vi "aptControl.vi"() -> (0 "Moving":bool, 3 "Current Position":sgl)   [LabVIEW 2010]
uses:
  <vilib>/DAQmx/write.llb/DAQmx Write (Digital 1D Bool 1Chan 1Samp).vi
  <vilib>/DAQmx/read.llb/DAQmx Read (Analog Wfm 1Chan NSamp).vi
  <vilib>/DAQmx/write.llb/DAQmx Write (Analog Wfm 1Chan NSamp).vi
  <vilib>/daqmx/miscellaneous.llb/DAQmx Fill In Error Info.vi
  <vilib>/Utility/file.llb/Write To Spreadsheet File (DBL).vi
  <vilib>/Utility/file.llb/Read From Spreadsheet File (DBL).vi
  <vilib>/gmath/NI_Gmath.lvlib
  <vilib>/Analysis/NI_AALBase.lvlib
panel:
  out "Scaner":string
  in  "Tab Control":enum32{"Control", "Curve", "Calibrate"}(tab)
  out "Es. Power (mW)":dbl format="%#.0f"
  in  "Possition (0:360)":dbl format="%#.2f"
  in  "Up":bool
  in  "Down":bool
  in  "Mirror\nOverride":bool
  in  "Galvo":bool=TRUE caption="AOD"
  in  "Lens":u16(ring)=10 items=["10X"=10, "20X"=20, "25X"=25, "16X"=16, "60X"=60]
  out "Out of range":bool
  in  "Home":bool
  in  "stop":bool
  out "Calibration Used":string
  out "Curve":cluster{"all rows":dbl[], "all rows":dbl[]}(graph)
  out "Curve 2":cluster{i32[], i32[]}(graph)
  in  "Start Calibration":bool
  in  "WaveLengths":dbl[](array[numeric])=[800.0, 890.0]
  out "Finished":bool
  in  "quit":bool
  out "Remaining min":dbl format="%#.2f"
  out "Acquiring":bool
  out "Waiting":bool
  out "Moving 2":bool
  in  "Repetitions":dbl=1.0
  in  "Step Size":dbl=4.0
  out "Current mW":dbl format="%#.0f"
  out "Old possition":sgl
  in  "MG17Motor 2":refnum<k7>(container)
  out "MinPos":sgl
  out "MaxPos":sgl
  in  "Target Position":dbl
  in  "MG17Motor":refnum<k7>(container)
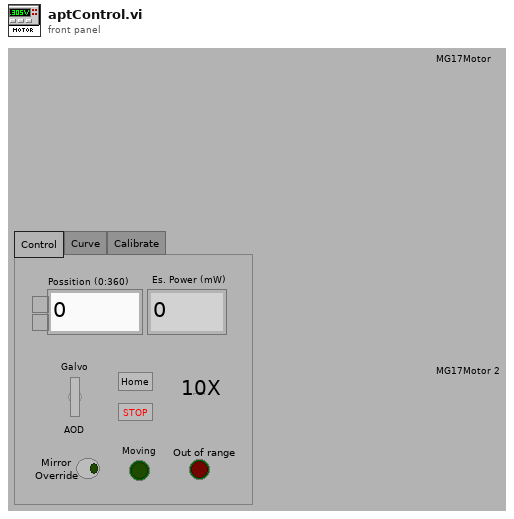
[diagram p1: front panel]
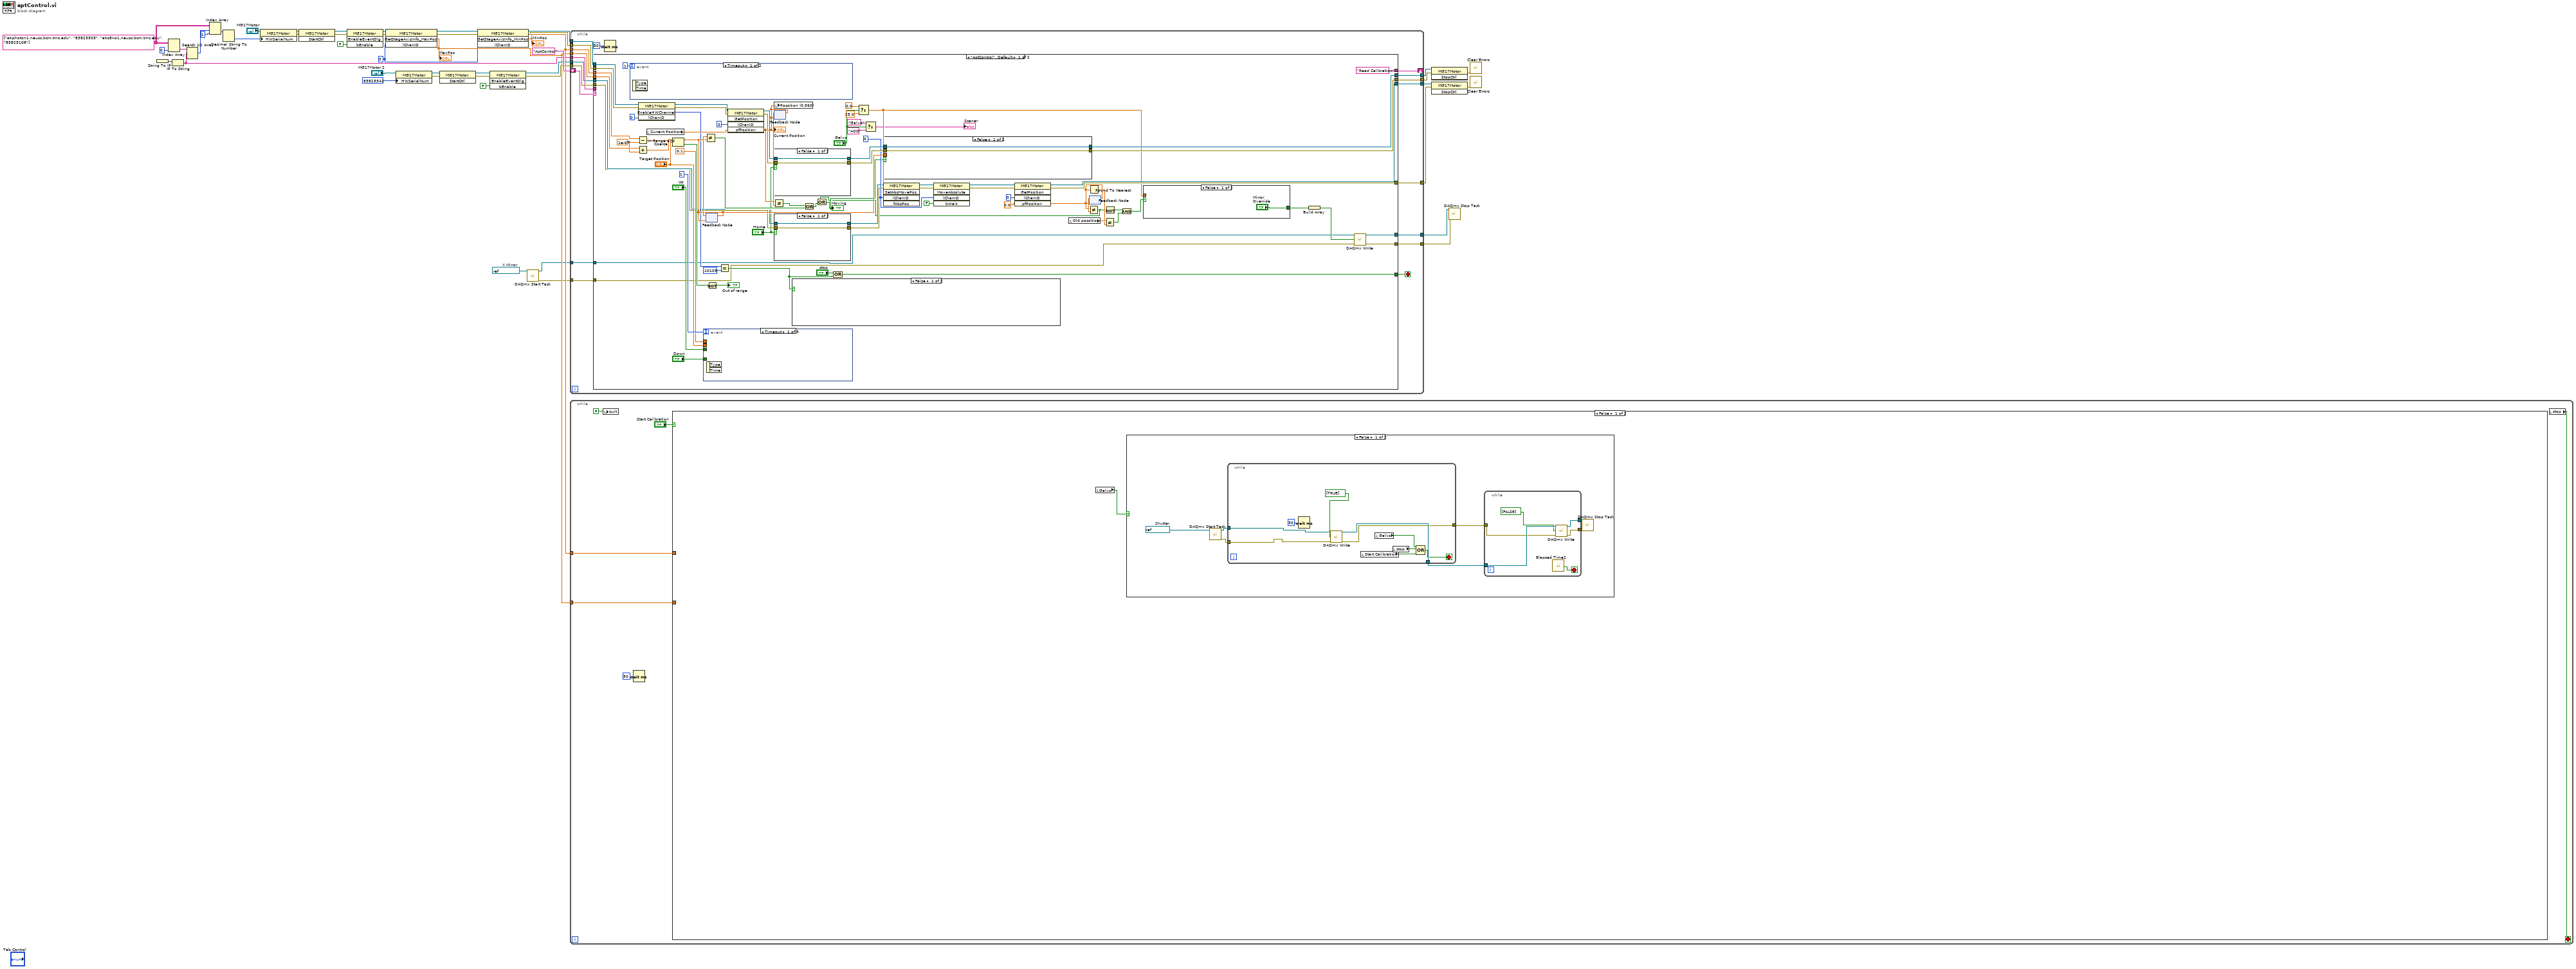
[diagram p0: block diagram]
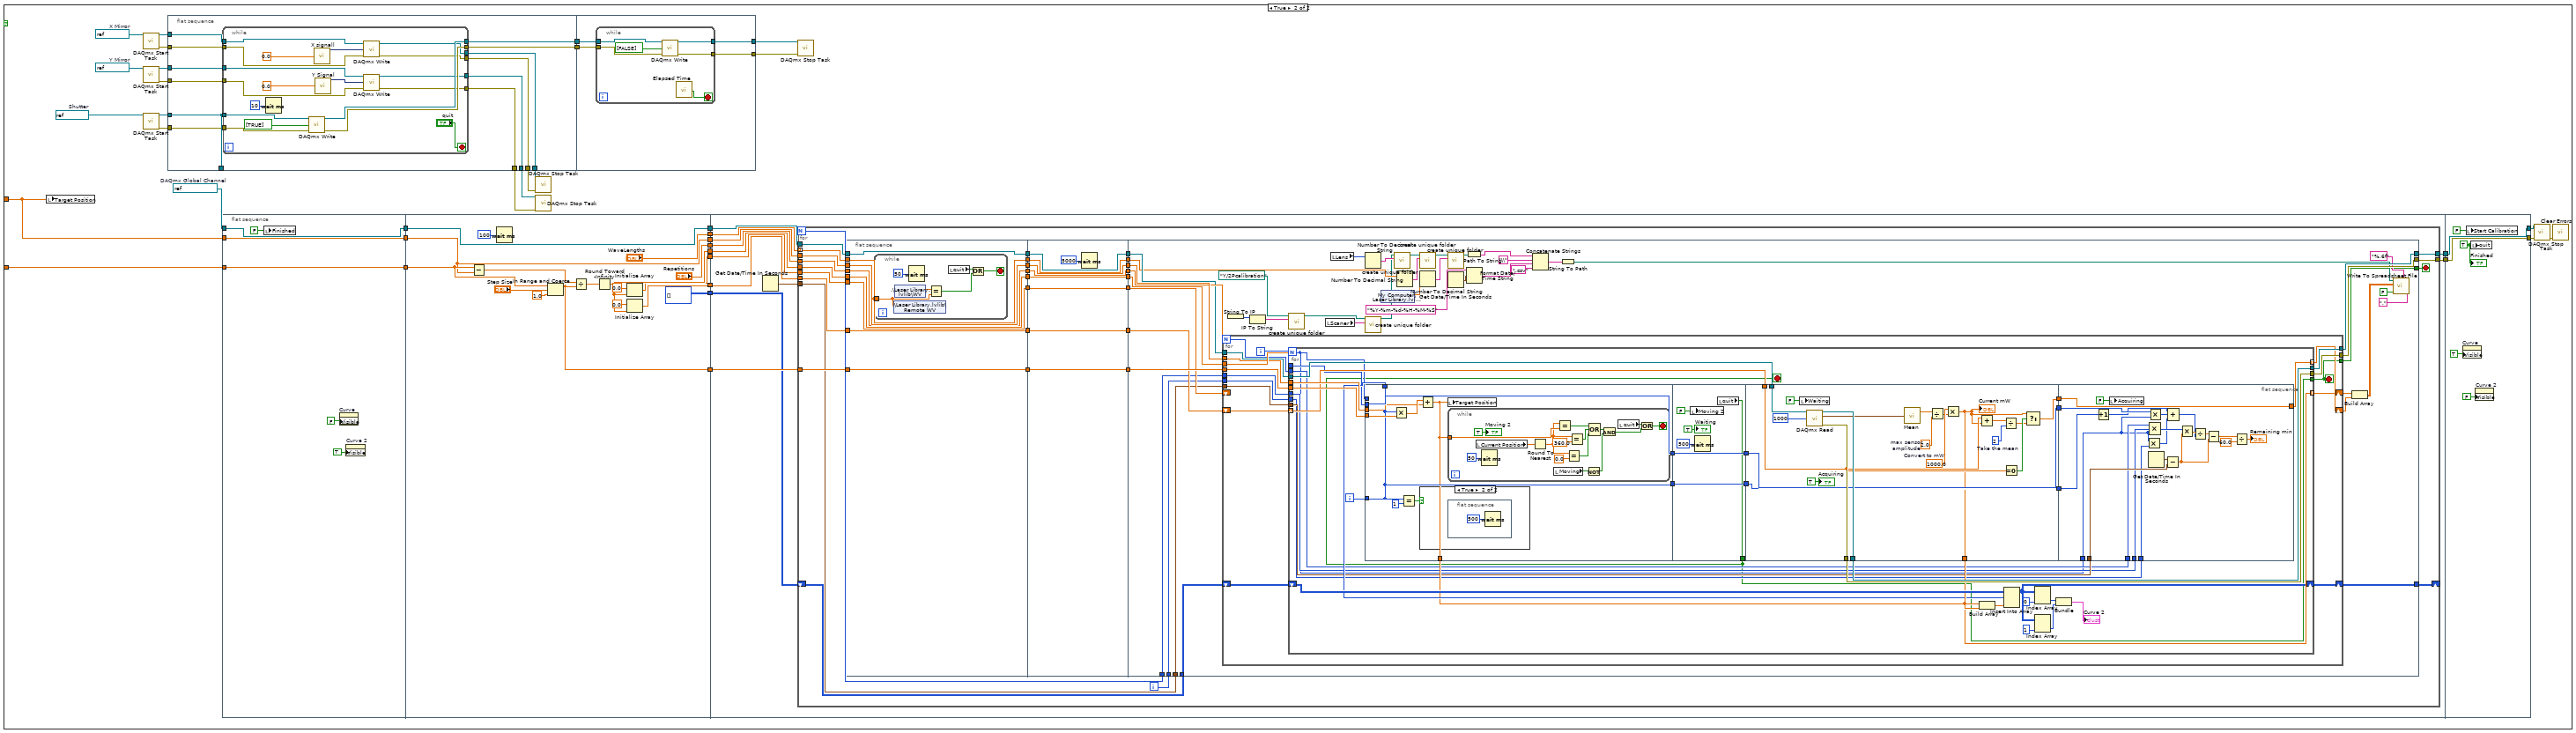
[diagram p3: hidden frame]
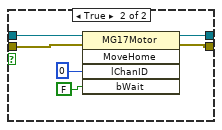
[diagram p5: hidden frame]
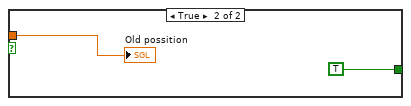
[diagram p6: hidden frame]
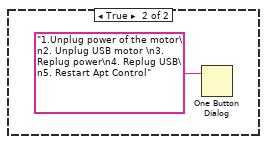
[diagram p7: hidden frame]
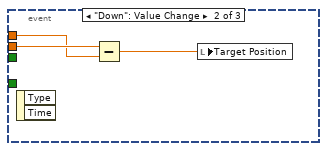
[diagram p8: hidden frame]
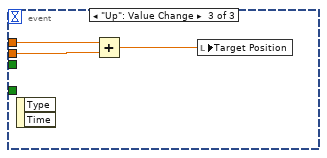
[diagram p9: hidden frame]
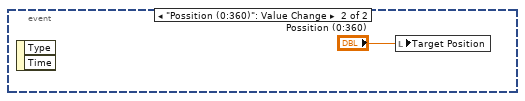
[diagram p10: hidden frame]
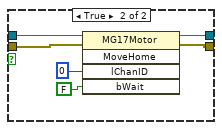
[diagram p11: hidden frame]
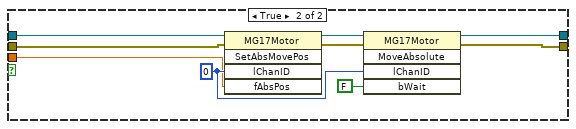
[diagram p12: hidden frame]
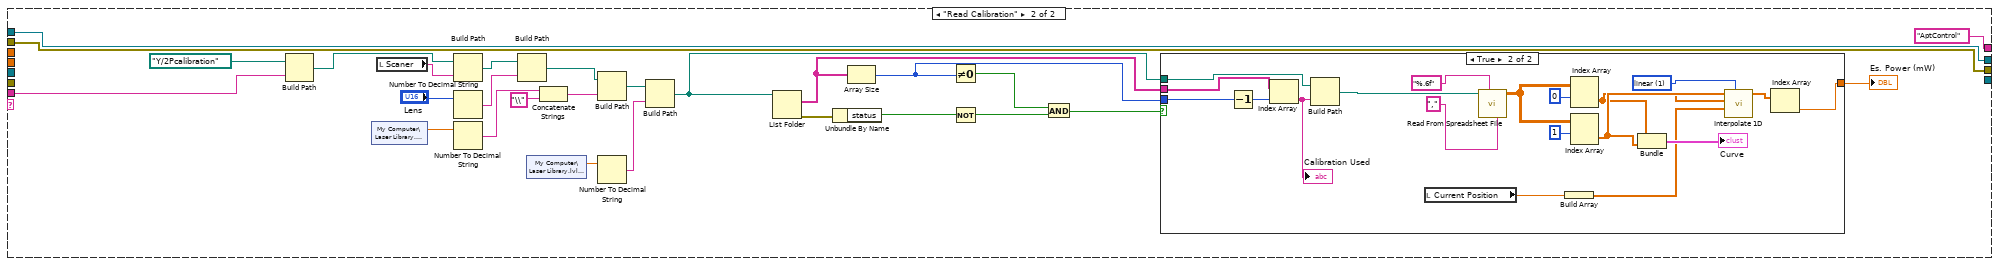
[diagram p13: hidden frame]
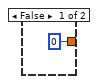
[diagram p14: hidden frame]
diagram:
  w5 = refnum<k21> "FlipMirror"  # X Mirror
  w31 = string[][] [["at-photon1.neusc.bcm.tmc.edu", "83823303"], ["at-s5no1.neusc.bcm.tmc.edu", "83823108"]]
  w41 = 0 ("lChanID")
  n1 = String To IP() -> (0:w35:u32)  [unwired: 1 in]
  n2 = Index Array(array=w31, index (col)=0 ("disabled index (col)")) -> (element=w33:string[])  [unwired: 1 in]
  n3 = IP To String(2:w35) -> (0:w27:string)  [unwired: 1 in]
  n4 = Search 1D Array(1D array=w33, element=w27) -> (index of element=w30:i32)  [unwired: 1 in]
  n5 = Index Array(array=w31, index (row)=w30, index (col)=1 ("disabled index (col)")) -> (element=w29:string)
  n6 = Decimal String To Number(string=w29) -> (number=w28:i32)  [unwired: 2 in, 1 out]
  n7 = property class="MG17Motor"(reference="MG17Motor", "HWSerialNum"=w28) -> (reference out=w44:refnum<k7>, error out=w43:errorcluster)  [unwired: 1 in]
  n8 = invoke class="MG17Motor" method="StartCtrl"(reference=w44, error in=w43) -> (reference out=w23:refnum<k7>, error out=w22:errorcluster)  [unwired: 1 in, 1 out]
  n9 = invoke class="MG17Motor" method="EnableEventDlg"(reference=w23, error in=w22, "bEnable"=FALSE) -> (reference out=w21:refnum<k7>, error out=w20:errorcluster)  [unwired: 1 in, 2 out]
  n10 = invoke class="MG17Motor" method="GetStageAxisInfo_MaxPos"(reference=w21, error in=w20, "lChanID"=w41) -> (reference out=w26:refnum<k7>, error out=w25:errorcluster, "GetStageAxisInfo_MaxPos"=w6:sgl)  [unwired: 1 in, 1 out]
  "MaxPos" <- w6
  n11 = property class="MG17Motor"(reference="MG17Motor 2", "HWSerialNum"=83823342) -> (reference out=w15:refnum<k7>, error out=w16:errorcluster)  [unwired: 1 in]
  n12 = invoke class="MG17Motor" method="StartCtrl"(reference=w15, error in=w16) -> (reference out=w18:refnum<k7>, error out=w19:errorcluster)  [unwired: 1 in, 1 out]
  n13 = invoke class="MG17Motor" method="GetStageAxisInfo_MinPos"(reference=w26, error in=w25, "lChanID"=w41) -> (reference out=w42:refnum<k7>, error out=w37:errorcluster, "GetStageAxisInfo_MinPos"=w7:sgl)  [unwired: 1 in, 1 out]
  "MinPos" <- w7
  n14 = invoke class="MG17Motor" method="EnableEventDlg"(reference=w18, error in=w19, "bEnable"=FALSE) -> (reference out=w13:refnum<k7>, error out=w8:errorcluster)  [unwired: 1 in, 2 out]
  n15 = call <vilib>:"DAQmx Start Task.vi"("task/channels in"=w5) -> ("task out"=w2:refnum<k21>, "error out"=w1:errorcluster)  [unwired: 13 in]
  n16 = while {
    tunnel: w42 -> [w64]
    tunnel: w6 -> [w62]
    tunnel: w7 -> [w61]
    tunnel: [w59] -> w40
    tunnel: [w60] -> w39
    tunnel: w37 -> [w58]
    shift-right: [w55] -> _
    shift-left: "AptControl" -> [w56]
    tunnel: w27 -> [w54]
    tunnel: w13 -> [w53]
    tunnel: [w52] -> w10
    tunnel: [w51] -> w9
    tunnel: w8 -> [w50]
    tunnel: [w49] -> w4
    tunnel: [w48] -> w3
    tunnel: w2 -> [w47]
    tunnel: w1 -> [w46]
    stop <- w57 stop-if-true
    n17 = case shown="\"AptControl\", Default" w56 {
      tunnel: w64 -> [w109 w204]
      tunnel: w62 -> [w118 _]
      tunnel: w61 -> [w119 _]
      tunnel: [w129 w204] -> w60
      tunnel: [w128 w203] -> w59
      tunnel: w58 -> [w108 w203]
      tunnel: [w122 _] -> w57
      tunnel: ["Read Calibration" "AptControl"] -> w55
      tunnel: w54 -> [_ w199]
      tunnel: w53 -> [w79 _]
      tunnel: [w94 _] -> w52
      tunnel: [w93 _] -> w51
      tunnel: w50 -> [w76 _]
      tunnel: [w71 _] -> w49
      tunnel: [w70 _] -> w48
      tunnel: w47 -> [w69 _]
      tunnel: w46 -> [w68 _]
      frame "AptControl", Default {
        w102 = 0 ("lChanID")
        w131 = 1e-07
        n18 = event shown="[0] Timeout" {
          selector: _ -> [_ _]
          dyn-events: _ -> [_ _]
          timeout: 1 -> [_ _]
          event Timeout {
            n19 = event-data() -> ()  [unwired: 1 in, 2 out]
          }
          event "Possition (0:360)": Value Change {
            n20 = event-data() -> ()  [unwired: 1 in, 2 out]
            n21 = local write "Target Position"("Possition (0:360)") -> ()
          }
        }
        n22 = Subtract(x=w119, y=w131) -> (x-y=w130:dbl)
        n23 = Add(x=w118, y=w131) -> (x+y=w132:dbl)
        n24 = invoke class="MG17Motor" method="EnableHWChannel"(reference=w109, error in=w108, "lChanID"=0) -> (reference out=w107:refnum<k7>, error out=w106:errorcluster, "EnableHWChannel"=w105:i32)  [unwired: 1 in, 1 out]
        n25 = local read "Current Position"() -> (w113:sgl)
        n26 = In Range and Coerce(upper limit=w132, x="Target Position", lower limit=w130) -> (coerced(x)=w135:dbl, In Range?=w134:bool)
        n27 = event shown="[0] Timeout" {
          selector: _ -> [_ _ _]
          dyn-events: _ -> [_ _ _]
          timeout: 1 -> [_ _ _]
          tunnel: "Up" -> [_ _ _]
          tunnel: "Down" -> [_ _ _]
          tunnel: 0.1 -> [_ w154 w158]
          tunnel: "Target Position" -> [_ w155 w157]
          event Timeout {
            n28 = event-data() -> ()  [unwired: 1 in, 2 out]
          }
          event "Down": Value Change {
            n29 = event-data() -> ()  [unwired: 1 in, 2 out]
            n30 = Subtract(x=w155, y=w154) -> (x-y=w153:dbl)
            n31 = local write "Target Position"(w153) -> ()
          }
          event "Up": Value Change {
            n32 = event-data() -> ()  [unwired: 1 in, 2 out]
            n33 = Add(x=w158, y=w157) -> (x+y=w156:dbl)
            n34 = local write "Target Position"(w156) -> ()
          }
        }
        n35 = feedback #1(w135) -> (w139:dbl)
        n36 = Not Equal?(x=w139, y=w135) -> (x != y?=w138:bool)
        n37 = feedback-in #1(w135) -> ()
        n38 = Not(x=w134) -> (.not. x?=→"Out of range":bool)
        n39 = Equal?(x=w105, y=10109) -> (x = y?=w104:bool)
        n40 = invoke class="MG17Motor" method="GetPosition"(reference=w107, error in=w106, "lChanID"=0, "pfPosition"=w113) -> (reference out=w127:refnum<k7>, error out=w111:errorcluster, "pfPosition"=w121:sgl)  [unwired: 1 in, 2 out]
        "Current Position" <- w121
        n41 = local write "Possition (0:360)"(w121) -> ()
        n42 = feedback #2(w121) -> (w137:sgl)
        n43 = Not Equal?(x=w121, y=w137) -> (x != y?=w136:bool)
        n44 = feedback-in #2(w121) -> ()
        n45 = case shown="False" "Home" {
          tunnel: w127 -> [w161 w167]
          tunnel: w111 -> [w160 w164]
          tunnel: [w161 w163] -> w126
          tunnel: [w160 w162] -> w125
          frame False {
          }
          frame True {
            n46 = invoke class="MG17Motor" method="MoveHome"(reference=w167, error in=w164, "lChanID"=0, "bWait"=FALSE) -> (reference out=w163:refnum<k7>, error out=w162:errorcluster)  [unwired: 1 in, 3 out]
          }
        }
        n47 = case shown="False" "Home" {
          tunnel: [w141 w146] -> w78
          tunnel: [w142 w145] -> w77
          tunnel: w79 -> [w141 w144]
          tunnel: w76 -> [w142 w143]
          frame False {
          }
          frame True {
            n48 = invoke class="MG17Motor" method="MoveHome"(reference=w144, error in=w143, "lChanID"=0, "bWait"=FALSE) -> (reference out=w146:refnum<k7>, error out=w145:errorcluster)  [unwired: 1 in, 3 out]
          }
        }
        n49 = case shown="False" w104 {
          frame False {
          }
          frame True {
            n50 = One Button Dialog(message="1.Unplug power of the motor\n2. Unplug USB motor \n3. Replug power\n4. Replug USB\n5. Restart Apt Control") -> ()  [unwired: 1 in, 1 out]
          }
        }
        n51 = Or(x=w136, y=w138) -> (x .or. y?=w67:bool)
        n52 = Compound Arithmetic op=OR("stop", w104) -> (w122:bool)
        n53 = Select(t=sgl 0.0 ("pfPosition"), s="Galvo", f=sgl 25.0 ("pfPosition")) -> (s? t:f=w91:sgl)
        n54 = Select(t="Galvo", s="Galvo", f="AOD") -> (s? t:f=→"Scaner":string)
        n55 = invoke class="MG17Motor" method="SetAbsMovePos"(reference=w78, error in=w77, "lChanID"=w102, "fAbsPos"=w91) -> (reference out=w100:refnum<k7>, error out=w103:errorcluster)  [unwired: 1 in, 3 out]
        n56 = invoke class="MG17Motor" method="MoveAbsolute"(reference=w100, error in=w103, "lChanID"=w102, "bWait"=FALSE) -> (reference out=w96:refnum<k7>, error out=w95:errorcluster)  [unwired: 1 in, 3 out]
        n57 = invoke class="MG17Motor" method="GetPosition"(reference=w96, error in=w95, "lChanID"=0, "pfPosition"=sgl 0.0) -> (reference out=w94:refnum<k7>, error out=w93:errorcluster, "pfPosition"=w86:sgl)  [unwired: 1 in, 2 out]
        n58 = local read "Old possition"() -> (w88:sgl)
        n59 = Round To Nearest(number=w86) -> (nearest integer value=w87:sgl)
        n60 = feedback #3(w86) -> (w92:sgl)
        n61 = Not Equal?(x=w86, y=w92) -> (x != y?=w65:bool)
        n62 = Or(x=w65, y=w67) -> (x .or. y?=w66:bool)
        "Moving" <- w66
        n63 = case shown="False" w66 {
          tunnel: w126 -> [w168 w178]
          tunnel: w135 -> [_ w174]
          tunnel: w125 -> [w169 w173]
          tunnel: [w169 w171] -> w128
          tunnel: [w168 w170] -> w129
          frame False {
          }
          frame True {
            w175 = 0 ("lChanID")
            n64 = invoke class="MG17Motor" method="SetAbsMovePos"(reference=w178, error in=w173, "lChanID"=w175, "fAbsPos"=w174) -> (reference out=w177:refnum<k7>, error out=w172:errorcluster)  [unwired: 1 in, 3 out]
            n65 = invoke class="MG17Motor" method="MoveAbsolute"(reference=w177, error in=w172, "lChanID"=w175, "bWait"=FALSE) -> (reference out=w170:refnum<k7>, error out=w171:errorcluster)  [unwired: 1 in, 3 out]
          }
        }
        n66 = feedback-in #3(w86) -> ()
        n67 = Not Equal?(x=w88, y=w87) -> (x != y?=w85:bool)
        n68 = Not(x=w65) -> (.not. x?=w90:bool)
        n69 = And(x=w90, y=w85) -> (x .and. y?=w89:bool)
        n70 = case shown="False" w89 {
          tunnel: w91 -> [_ w151]
          tunnel: ["Mirror\nOverride" TRUE] -> w84
          frame False {
          }
          frame True {
            "Old possition" <- w151
          }
        }
        n71 = Build Array(w84) -> (w72:bool[])
        n72 = call-poly <vilib>:"DAQmx Write.vi"("task/channels in"=w69, "data"=w72, "error in"=w68) -> ("task out"=w71:refnum<k21>, "error out"=w70:errorcluster)  [unwired: 10 in, 1 out]
      }
      frame "Read Calibration" {
        n73 = Build Path(base path=path "Y:/2Pcalibration", name or relative path=w199) -> (appended path=w186:path)
        n74 = shared-variable "My Computer\\Laser Library.lvlib\\WV"() -> (w189:dbl)  [unwired: 1 in, 1 out]
        n75 = local read "Scaner"() -> (w179:string)
        n76 = Build Path(base path=w186, name or relative path=w179) -> (appended path=w187:path)
        n77 = Number To Decimal String(number="Lens") -> (decimal integer string=w201:string)  [unwired: 1 in]
        n78 = Number To Decimal String(number=w189) -> (decimal integer string=w188:string)  [unwired: 1 in]
        n79 = Build Path(base path=w187, name or relative path=w201) -> (appended path=w183:path)
        n80 = shared-variable "My Computer\\Laser Library.lvlib\\GDD"() -> (w185:dbl)  [unwired: 1 in, 1 out]
        n81 = Concatenate Strings(w188, "\\" ("string")) -> (w196:string)
        n82 = Build Path(base path=w183, name or relative path=w196) -> (appended path=w182:path)
        n83 = Number To Decimal String(number=w185) -> (decimal integer string=w184:string)  [unwired: 1 in]
        n84 = Build Path(base path=w182, name or relative path=w184) -> (appended path=w181:path)
        n85 = List Folder(path=w181) -> (filenames=w200:string[], error out=w195:errorcluster)  [unwired: 3 in, 2 out]
        n86 = Unbundle By Name(w195) -> ("status"=w191:bool)
        n87 = Array Size(array=w200) -> (size(s)=w198:i32)
        n88 = Not Equal To 0?(x=w198) -> (x != 0?=w192:bool)
        n89 = Not(x=w191) -> (.not. x?=w190:bool)
        n90 = And(x=w192, y=w190) -> (x .and. y?=w194:bool)
        n91 = case shown="True" w194 {
          tunnel: w200 -> [_ w225]
          tunnel: w198 -> [_ w224]
          tunnel: w181 -> [_ w222]
          tunnel: [0 w211] -> w193
          frame False {
          }
          frame True {
            w213 = 1 items=["nearest", "linear", "spline", "cubic Hermite", "Lagrange"] ("method")
            n92 = Decrement(x=w224) -> (x-1=w223:i32)
            n93 = Index Array(array=w225, index=w223) -> (element=w221:string)
            "Calibration Used" <- w221
            n94 = Build Path(base path=w222, name or relative path=w221) -> (appended path=w220:path)
            n95 = local read "Current Position"() -> (w219:sgl)
            n96 = call-poly <vilib>:"Read From Spreadsheet File.vi"("delimiter (\\t)"="," ("delimiter (\\t)"), "format (%.3f)"="%.6f", "file path (dialog if empty)"=w220) -> ("all rows"=w218:dbl[][])  [unwired: 4 in, 4 out]
            n97 = Build Array(w219) -> (w209:sgl[])
            n98 = Index Array(array=w218, index (row)=0 ("disabled index (col)")) -> (element=w207:dbl[])  [unwired: 1 in]
            n99 = Index Array(array=w218, index (row)=1 ("disabled index (col)")) -> (element=w208:dbl[])  [unwired: 1 in]
            n100 = Bundle("all rows"=w207, "all rows"=w208) -> (→"Curve":cluster{"all rows":dbl[], "all rows":dbl[]})  [unwired: 1 in]
            n101 = call <vilib>:"Interpolate 1D.vi"("method"=w213, "xi"=w209, "X"=w207, "Y"=w208) -> ("yi"=w212:dbl[])  [unwired: 5 in, 2 out]
            n102 = Index Array(array=w212) -> (element=w211:dbl)  [unwired: 1 in]
          }
        }
        "Es. Power (mW)" <- w193
      }
    }
    n103 = Wait (ms)(milliseconds to wait=u32 50) -> ()  [unwired: 1 out]
  }
  n104 = while {
    tunnel: w7 -> [w231]
    tunnel: w6 -> [w230]
    stop <- w228 stop-if-true
    n105 = local write "quit"(FALSE) -> ()
    n106 = Wait (ms)(milliseconds to wait=u32 50) -> ()  [unwired: 1 out]
    n107 = case shown="False" "Start Calibration" {
      tunnel: w230 -> [_ w257]
      tunnel: w231 -> [_ w256]
      frame False {
        n108 = local read "Galvo"() -> (w232:bool)
        n109 = case shown="False" w232 {
          frame False {
            w239 = refnum<k21> "Shutter"  # Shutter
            n110 = call <vilib>:"DAQmx Start Task.vi"("task/channels in"=w239) -> ("task out"=w238:refnum<k21>, "error out"=w237:errorcluster)  [unwired: 13 in]
            n111 = while {
              tunnel: w238 -> [w254]
              tunnel: w237 -> [w253]
              tunnel: [w252] -> w236
              tunnel: [w251] -> w235
              stop <- w248 stop-if-true
              n112 = Wait (ms)(milliseconds to wait=u32 30) -> ()  [unwired: 1 out]
              n113 = call-poly <vilib>:"DAQmx Write.vi"("task/channels in"=w254, "data"=bool[] [TRUE], "error in"=w253) -> ("task out"=w252:refnum<k21>, "error out"=w251:errorcluster)  [unwired: 10 in, 1 out]
              n114 = local read "Start Calibration"() -> (w249:bool)
              n115 = local read "Galvo"() -> (w246:bool)
              n116 = local read "stop"() -> (w250:bool)
              n117 = Compound Arithmetic op=OR(w246, w250, w249) -> (w248:bool)
            }
            n118 = while {
              tunnel: w236 -> [w245]
              tunnel: w235 -> [w244]
              tunnel: [w243] -> w234
              tunnel: [w242] -> w233
              stop <- w240 stop-if-true
              n119 = call "Elapsed Time2"() -> ("Time has Elapsed"=w240:bool)  [unwired: 12 in, 7 out]
              n120 = call-poly <vilib>:"DAQmx Write.vi"("task/channels in"=w245, "data"=bool[] [FALSE], "error in"=w244) -> ("task out"=w243:refnum<k21>, "error out"=w242:errorcluster)  [unwired: 10 in, 1 out]
            }
            n121 = call <vilib>:"DAQmx Stop Task.vi"("task/channels in"=w234, "error in"=w233) -> ()  [unwired: 12 in, 2 out]
          }
          frame True {
          }
        }
      }
      frame True {
        w264 = refnum<k21> "Y Mirror"  # Y Mirror
        w265 = refnum<k21> "X Mirror"  # X Mirror
        w266 = refnum<k21> "Shutter"  # Shutter
        w273 = refnum<k21> "PowerMeter"  # DAQmx Global Channel
        n122 = local write "Target Position"(w256) -> ()
        n123 = call <vilib>:"DAQmx Start Task.vi"("task/channels in"=w265) -> ("task out"=w261:refnum<k21>, "error out"=w259:errorcluster)  [unwired: 13 in]
        n124 = call <vilib>:"DAQmx Start Task.vi"("task/channels in"=w264) -> ("task out"=w263:refnum<k21>, "error out"=w258:errorcluster)  [unwired: 13 in]
        n125 = call <vilib>:"DAQmx Start Task.vi"("task/channels in"=w266) -> ("task out"=w262:refnum<k21>, "error out"=w260:errorcluster)  [unwired: 13 in]
        n126 = flat-sequence {
          tunnel: [w296] -> _
          tunnel: w261 -> [w304]
          tunnel: [w303] -> w278
          tunnel: [w302] -> w277
          tunnel: [w301] -> w270
          tunnel: [w300] -> w269
          tunnel: [w299] -> w268
          tunnel: [w298] -> w267
          tunnel: w263 -> [w297]
          tunnel: w262 -> [w296]
          tunnel: w260 -> [w295]
          tunnel: w259 -> [w294]
          tunnel: w258 -> [w293]
          tunnel: w278 -> [w327]
          tunnel: [w326] -> w272
          tunnel: [w325] -> w271
          tunnel: w277 -> [w324]
          frame #0 {
            n127 = while {
              tunnel: w296 -> [w318]
              tunnel: w304 -> [w320]
              tunnel: w297 -> [w319]
              tunnel: [w316] -> w303
              tunnel: [w315] -> w302
              tunnel: [w312] -> w301
              tunnel: [w311] -> w300
              tunnel: [w310] -> w299
              tunnel: [w309] -> w298
              tunnel: w295 -> [w308]
              tunnel: w294 -> [w307]
              tunnel: w293 -> [w306]
              stop <- "quit" stop-if-true
              n128 = Wait (ms)(milliseconds to wait=u32 10) -> ()  [unwired: 1 out]
              n129 = call-poly <vilib>:"DAQmx Write.vi"("task/channels in"=w318, "data"=bool[] [TRUE], "error in"=w308) -> ("task out"=w316:refnum<k21>, "error out"=w315:errorcluster)  [unwired: 10 in, 1 out]
              n130 = call "X signall"("Amplitude"=0.0) -> ("Sine"=w314:dynamicdata)  [unwired: 13 in, 1 out]
              n131 = call "Y Signal"("Amplitude"=0.0) -> ("Sine"=w313:dynamicdata)  [unwired: 13 in, 1 out]
              n132 = call-poly <vilib>:"DAQmx Write.vi"("task/channels in"=w320, "data"=w314, "error in"=w307) -> ("task out"=w312:refnum<k21>, "error out"=w311:errorcluster)  [unwired: 10 in, 1 out]
              n133 = call-poly <vilib>:"DAQmx Write.vi"("task/channels in"=w319, "data"=w313, "error in"=w306) -> ("task out"=w310:refnum<k21>, "error out"=w309:errorcluster)  [unwired: 10 in, 1 out]
            }
          }
          frame #1 {
            n134 = while {
              tunnel: w327 -> [w332]
              tunnel: [w330] -> w326
              tunnel: [w329] -> w325
              tunnel: w324 -> [w328]
              stop <- w333 stop-if-true
              n135 = call-poly <vilib>:"DAQmx Write.vi"("task/channels in"=w332, "data"=bool[] [FALSE], "error in"=w328) -> ("task out"=w330:refnum<k21>, "error out"=w329:errorcluster)  [unwired: 10 in, 1 out]
              n136 = call "Elapsed Time"() -> ("Time has Elapsed"=w333:bool)  [unwired: 12 in, 7 out]
            }
          }
        }
        n137 = flat-sequence {
          tunnel: w257 -> [w337]
          tunnel: w273 -> [w338]
          tunnel: w256 -> [w339]
          tunnel: [w339] -> w292
          tunnel: [w338] -> w291
          tunnel: [w337] -> w290
          tunnel: [w353] -> w289
          tunnel: ["Repetitions"] -> w288
          tunnel: [w352] -> w287
          tunnel: [w356] -> w286
          tunnel: [w351] -> w285
          tunnel: [w350] -> w284
          tunnel: [i32[][] []] -> w283
          tunnel: ["WaveLengths"] -> w282
          tunnel: [w349] -> w281
          tunnel: w292 -> [w353]
          tunnel: w291 -> [w356]
          tunnel: w290 -> [w354]
          tunnel: w289 -> [w368]
          tunnel: w288 -> [w367]
          tunnel: w287 -> [w366]
          tunnel: w286 -> [w365]
          tunnel: w285 -> [w363]
          tunnel: w284 -> [w362]
          tunnel: w283 -> [w360]
          tunnel: w282 -> [w361]
          tunnel: w281 -> [w364]
          tunnel: [w359] -> w280
          tunnel: [w358] -> w279
          tunnel: [w594] -> w274
          tunnel: [w595] -> w275
          tunnel: w280 -> [w595]
          tunnel: w279 -> [w594]
          frame #0 {
            n138 = local write "Finished"(FALSE ("Finished")) -> ()
            n139 = property on="Curve" class="XYGraph (strict)"("Visible"=FALSE) -> ()  [unwired: 2 in, 2 out]
            n140 = property on="Curve 2" class="XYGraph (strict)"("Visible"=TRUE) -> ()  [unwired: 2 in, 2 out]
          }
          frame #1 {
            n141 = Subtract(x=w354, y=w353) -> (x-y=w344:sgl)
            n142 = Wait (ms)(milliseconds to wait=u32 100) -> ()  [unwired: 1 out]
            n143 = In Range and Coerce(upper limit=w354, x="Step Size", lower limit=1.0) -> (coerced(x)=w352:dbl)  [unwired: 1 out]
            n144 = Divide(x=w344, y=w352) -> (x/y=w345:dbl)
            n145 = Round Toward -Infinity(1:w345) -> (0:w351:dbl)
            n146 = Initialize Array(0.0 ("element"), w351) -> (w350:dbl[])
            n147 = Initialize Array(0.0 ("element"), w351) -> (w349:dbl[])
          }
          frame #2 {
            n148 = Get Date/Time In Seconds() -> (seconds since 1Jan1904=w357:timestamp)
            n149 = for {
              N -> [w371]
              tunnel: w368 -> [w400]
              tunnel: w367 -> [w399]
              tunnel: w366 -> [w398]
              tunnel: w365 -> [w397]
              tunnel: [w396] -> w359
              tunnel: [w395] -> w358
              tunnel: w364 -> [w394]
              tunnel: w363 -> [w393]
              tunnel: w362 -> [w392]
              tunnel: w361 -> [w391] mode=indexing
              shift-right: [w373] -> _
              shift-left: w360 -> [w374]
              tunnel: w357 -> [w372]
              i -> [w370]
              stop <- w369 stop-if-true
              n150 = flat-sequence {
                tunnel: w391 -> [w401]
                tunnel: w392 -> [w402]
                tunnel: w393 -> [w403]
                tunnel: w394 -> [w404]
                tunnel: w397 -> [w405]
                tunnel: w398 -> [w406]
                tunnel: w399 -> [w407]
                tunnel: w400 -> [w408]
                tunnel: [w408] -> w390
                tunnel: [w407] -> w388
                tunnel: [w406] -> w386
                tunnel: [w405] -> w384
                tunnel: [w404] -> w382
                tunnel: [w403] -> w380
                tunnel: [w402] -> w378
                tunnel: [w401] -> w376
                tunnel: w390 -> [w423]
                tunnel: [w423] -> w389
                tunnel: w388 -> [w422]
                tunnel: [w422] -> w387
                tunnel: w386 -> [w421]
                tunnel: [w421] -> w385
                tunnel: w384 -> [w420]
                tunnel: [w420] -> w383
                tunnel: w382 -> [w419]
                tunnel: [w419] -> w381
                tunnel: w380 -> [w418]
                tunnel: [w418] -> w379
                tunnel: w378 -> [w417]
                tunnel: [w417] -> w377
                tunnel: w376 -> [w416]
                tunnel: [w416] -> w375
                tunnel: [w465] -> w373
                tunnel: [w466] -> w395
                tunnel: [w467] -> w396
                tunnel: w370 -> [w434]
                tunnel: w371 -> [w435]
                tunnel: w372 -> [w436]
                tunnel: w374 -> [w437]
                tunnel: w375 -> [w438]
                tunnel: w377 -> [w458]
                tunnel: w379 -> [w459]
                tunnel: w381 -> [w460]
                tunnel: w383 -> [w461]
                tunnel: w385 -> [w462]
                tunnel: w387 -> [w463]
                tunnel: w389 -> [w464]
                tunnel: [w424] -> w369
                frame #0 {
                  n151 = while {
                    tunnel: w401 -> [w413]
                    stop <- w409 stop-if-true
                    n152 = shared-variable ".\\Laser Library.lvlib\\Remote WV"(w413) -> ()  [unwired: 1 in, 1 out]
                    n153 = shared-variable ".\\Laser Library.lvlib\\WV"() -> (w412:dbl)  [unwired: 1 in, 1 out]
                    n154 = Wait (ms)(milliseconds to wait=u32 50) -> ()  [unwired: 1 out]
                    n155 = Equal?(x=w412, y=w413) -> (x = y?=w410:bool)
                    n156 = local read "quit"() -> (w411:bool)
                    n157 = Or(x=w411, y=w410) -> (x .or. y?=w409:bool)
                  }
                }
                frame #1 {
                  n158 = Wait (ms)(milliseconds to wait=u32 5000) -> ()  [unwired: 1 out]
                }
                frame #2 {
                  n159 = for {
                    N: w463 -> [w470]
                    tunnel: w459 -> [w484]
                    tunnel: w464 -> [w483]
                    tunnel: w462 -> [w482]
                    tunnel: w461 -> [w481]
                    tunnel: [w480] -> w467
                    tunnel: [w479] -> w466
                    shift-right: [w478] -> w440
                    shift-left: w460 -> [w476]
                    shift-right: [w477] -> w441
                    shift-left: w458 -> [_]
                    shift-right: [w475] -> w465
                    shift-left: w437 -> [w474]
                    tunnel: w436 -> [w472]
                    tunnel: w435 -> [w471]
                    tunnel: w434 -> [w469]
                    tunnel: [w468] -> w424
                    i -> [w473]
                    stop <- w468 stop-if-true
                    n160 = for {
                      N: w484 -> [w488]
                      tunnel: w483 -> [w517]
                      tunnel: w482 -> [w516]
                      tunnel: w481 -> [w514]
                      tunnel: [w513] -> w480
                      tunnel: [w512] -> w479
                      tunnel: [w487] -> w478 mode=indexing
                      tunnel: w476 -> [w509] mode=indexing
                      tunnel: [w505] -> w477 mode=indexing
                      shift-right: [w502] -> w475
                      shift-left: w474 -> [w510]
                      tunnel: w473 -> [w499]
                      tunnel: w472 -> [w498]
                      tunnel: w471 -> [w497]
                      tunnel: w470 -> [w496]
                      tunnel: w469 -> [w495]
                      tunnel: [w486] -> w468
                      i -> [w515]
                      stop <- w486 stop-if-true
                      n161 = flat-sequence {
                        tunnel: w515 -> [w521]
                        tunnel: w516 -> [w525]
                        tunnel: w517 -> [w522]
                        tunnel: [w518] -> w505
                        tunnel: [w521] -> w506
                        tunnel: w499 -> [w524]
                        tunnel: [w524] -> w492
                        tunnel: [w521] -> w489
                        tunnel: w488 -> [_]
                        tunnel: [w547] -> w493
                        tunnel: w492 -> [w547]
                        tunnel: [w546] -> w490
                        tunnel: w489 -> [w546]
                        tunnel: [w543] -> w486
                        tunnel: w514 -> [w568]
                        tunnel: [w567] -> w513
                        tunnel: [w566] -> w512
                        tunnel: w509 -> [w552]
                        tunnel: [w560] -> w511
                        tunnel: [w549] -> w508
                        tunnel: [w554] -> w494
                        tunnel: w493 -> [w554]
                        tunnel: [w553] -> w491
                        tunnel: w490 -> [w553]
                        tunnel: w511 -> [w583]
                        tunnel: w498 -> [w588]
                        tunnel: w497 -> [w587]
                        tunnel: w496 -> [w586]
                        tunnel: w488 -> [w575]
                        tunnel: w495 -> [w576]
                        tunnel: w494 -> [w577]
                        tunnel: w491 -> [w585]
                        tunnel: [w583] -> w487
                        frame #0 {
                          n162 = Multiply(x=w521, y=w525) -> (x*y=w523:dbl)
                          n163 = Equal?(x=w521, y=1) -> (x = y?=w520:bool)
                          n164 = Add(x=w523, y=w522) -> (x+y=w518:dbl)
                          n165 = case shown="True" w520 {
                            frame False {
                            }
                            frame True {
                              n166 = flat-sequence {
                                frame #0 {
                                n167 = Wait (ms)(milliseconds to wait=u32 500) -> ()  [unwired: 1 out]
                                }
                              }
                            }
                          }
                          n168 = local write "Target Position"(w518) -> ()
                          n169 = while {
                            tunnel: w518 -> [w541]
                            stop <- w528 stop-if-true
                            n170 = local read "Current Position"() -> (w530:sgl)
                            n171 = Wait (ms)(milliseconds to wait=u32 50) -> ()  [unwired: 1 out]
                            n172 = Round To Nearest(number=w530) -> (nearest integer value=w535:sgl)
                            n173 = local read "Moving"() -> (w531:bool)
                            n174 = Equal?(x=w535, y=w541) -> (x = y?=w539:bool)
                            n175 = Equal?(x=w535, y=0.0) -> (x = y?=w536:bool)
                            n176 = Equal?(x=w535, y=360.0) -> (x = y?=w537:bool)
                            n177 = Not(x=w531) -> (.not. x?=w540:bool)
                            n178 = Compound Arithmetic op=OR(w539, w537, w536) -> (w538:bool)
                            n179 = And(x=w538, y=w540) -> (x .and. y?=w529:bool)
                            n180 = local read "quit"() -> (w527:bool)
                            n181 = Or(x=w527, y=w529) -> (x .or. y?=w528:bool)
                            "Moving 2" <- TRUE
                          }
                        }
                        frame #1 {
                          n182 = local write "Moving 2"(FALSE) -> ()
                          n183 = Wait (ms)(milliseconds to wait=u32 500) -> ()  [unwired: 1 out]
                          n184 = local read "quit"() -> (w543:bool)
                          "Waiting" <- TRUE
                        }
                        frame #2 {
                          w555 = 2.0  # max sensor  amplitude
                          w557 = 1000.0  # Convert to mW
                          w563 = 2  # Take the mean
                          n185 = local write "Waiting"(FALSE) -> ()
                          n186 = call-poly <vilib>:"DAQmx Read.vi"("task/channels in"=w568, "number of samples per channel"=1000) -> ("task out"=w567:refnum<k21>, "data"=w558:waveform(dbl), "error out"=w566:errorcluster)  [unwired: 1 in, 10 out]
                          n187 = call <vilib>:"Mean.vi"("X"=w558) -> ("mean"=w559:dbl)  [unwired: 1 out]
                          n188 = Divide(x=w559, y=w555) -> (x/y=w556:dbl)
                          n189 = Multiply(x=w557, y=w556) -> (x*y=w549:dbl)
                          "Current mW" <- w549
                          n190 = Add(x=w552, y=w549) -> (x+y=w562:dbl)
                          n191 = Divide(x=w562, y=w563) -> (x/y=w561:dbl)
                          n192 = Equal To 0?(x=w552) -> (x = 0?=w564:bool)
                          n193 = Select(t=w549, s=w564, f=w561) -> (s? t:f=w560:dbl)
                          "Acquiring" <- TRUE ("Acquiring")
                        }
                        frame #3 {
                          n194 = Increment(x=w585) -> (x+1=w574:i32)
                          n195 = local write "Acquiring"(FALSE ("Acquiring")) -> ()
                          n196 = Multiply(x=w575, y=w576) -> (x*y=w572:i32)
                          n197 = Multiply(x=w577, y=w575) -> (x*y=w573:i32)
                          n198 = Get Date/Time In Seconds() -> (seconds since 1Jan1904=w589:timestamp)
                          n199 = Compound Arithmetic op=MULTIPLY(w586, w587, w575) -> (w582:i32)
                          n200 = Subtract(x=w589, y=w588) -> (x-y=w580:dbl)
                          n201 = Compound Arithmetic op=ADD(w574, w573, w572) -> (w571:i32)
                          n202 = Multiply(x=w582, y=w580) -> (x*y=w581:dbl)
                          n203 = Divide(x=w581, y=w571) -> (x/y=w579:dbl)
                          n204 = Subtract(x=w579, y=w580) -> (x-y=w578:dbl)
                          n205 = Divide(x=w578, y=60.0) -> (x/y=→"Remaining min":dbl)
                        }
                      }
                      n206 = Build Array(w505, w508) -> (w507:dbl[])
                      n207 = Insert Into Array(array=w510, index (row)=w506, new element=w507) -> (w502:i32[][])  [unwired: 1 in]
                      n208 = Index Array(array=w502, index (col)=0 ("index")) -> (element=w503:i32[])  [unwired: 1 in]
                      n209 = Index Array(array=w502, index (col)=1 ("index")) -> (element=w500:i32[])  [unwired: 1 in]
                      n210 = Bundle(w503, w500) -> (→"Curve 2":cluster{i32[], i32[]})  [unwired: 1 in]
                    }
                  }
                  n211 = String To IP() -> (0:w451:u32)  [unwired: 1 in]
                  n212 = IP To String(2:w451) -> (0:w433:string)  [unwired: 1 in]
                  n213 = call "create unique folder.vi"("string"=w433, "path 2"=path "Y:/2Pcalibration") -> ("path"=w432:path)  [unwired: 9 in]
                  n214 = local read "Scaner"() -> (w425:string)
                  n215 = local read "Lens"() -> (w426:u16)
                  n216 = Number To Decimal String(number=w426) -> (decimal integer string=w442:string)  [unwired: 1 in]
                  n217 = call "create unique folder.vi"("string"=w425, "path 2"=w432) -> ("path"=w431:path)  [unwired: 9 in]
                  n218 = shared-variable "My Computer\\Laser Library.lvlib\\GDD"() -> (w430:dbl)  [unwired: 1 in, 1 out]
                  n219 = call "create unique folder.vi"("string"=w442, "path 2"=w431) -> ("path"=w443:path)  [unwired: 9 in]
                  n220 = Number To Decimal String(number=w438) -> (decimal integer string=w450:string)  [unwired: 1 in]
                  n221 = call "create unique folder.vi"("string"=w450, "path 2"=w443) -> ("path"=w429:path)  [unwired: 9 in]
                  n222 = Number To Decimal String(number=w430) -> (decimal integer string=w427:string)  [unwired: 1 in]
                  n223 = call "create unique folder.vi"("string"=w427, "path 2"=w429) -> ("path"=w428:path)  [unwired: 9 in]
                  n224 = Get Date/Time In Seconds() -> (seconds since 1Jan1904=w454:timestamp)
                  n225 = Path To String(path=w428) -> (string=w449:string)
                  n226 = Format Date/Time String(time format string (%c)="%Y-%m-%d-%H-%M-%S", seconds (now)=w454) -> (date/time string=w447:string)  [unwired: 1 in]
                  n227 = Concatenate Strings(w449, "\\" ("string"), w447, ".csv" ("string")) -> (w446:string)
                  n228 = String To Path(string=w446) -> (path=w445:path)
                  n229 = Build Array(w441, w440) -> (w439:dbl[][])
                  n230 = call-poly <vilib>:"Write To Spreadsheet File.vi"("delimiter (\\t)"="," ("delimiter (\\t)"), "format (%.3f)"="%.6f", "append to file? (new file:F)"=FALSE, "2D data"=w439, "file path (dialog if empty)"=w445) -> ()  [unwired: 2 in, 2 out]
                }
              }
            }
          }
          frame #3 {
            w593 = TRUE ("Finished")
            n231 = property on="Curve" class="XYGraph (strict)"("Visible"=TRUE) -> ()  [unwired: 2 in, 2 out]
            n232 = local write "Start Calibration"(FALSE) -> ()
            n233 = local write "quit"(w593) -> ()
            n234 = property on="Curve 2" class="XYGraph (strict)"("Visible"=FALSE) -> ()  [unwired: 2 in, 2 out]
            "Finished" <- w593
          }
        }
        n235 = call <vilib>:"DAQmx Stop Task.vi"("task/channels in"=w270, "error in"=w269) -> ()  [unwired: 12 in, 2 out]
        n236 = call <vilib>:"DAQmx Stop Task.vi"("task/channels in"=w268, "error in"=w267) -> ()  [unwired: 12 in, 2 out]
        n237 = call <vilib>:"DAQmx Stop Task.vi"("task/channels in"=w272, "error in"=w271) -> ()  [unwired: 12 in, 2 out]
        n238 = call <vilib>:"DAQmx Stop Task.vi"("task/channels in"=w275, "error in"=w274) -> ("error out"=w276:errorcluster)  [unwired: 13 out]
        n239 = call <vilib>:"Clear Errors.vi"("error in (no error)"=w276) -> ()  [unwired: 6 in, 1 out]
      }
    }
    n240 = local read "stop"() -> (w228:bool)
  }
  n241 = invoke class="MG17Motor" method="StopCtrl"(reference=w39, error in=w40) -> (error out=w38:errorcluster)  [unwired: 1 in, 2 out]
  n242 = invoke class="MG17Motor" method="StopCtrl"(reference=w10, error in=w9) -> (error out=w11:errorcluster)  [unwired: 1 in, 2 out]
  n243 = call <vilib>:"DAQmx Stop Task.vi"("task/channels in"=w4, "error in"=w3) -> ()  [unwired: 12 in, 2 out]
  n244 = call <vilib>:"Clear Errors.vi"("error in (no error)"=w38) -> ()  [unwired: 6 in, 1 out]
  n245 = call <vilib>:"Clear Errors.vi"("error in (no error)"=w11) -> ()  [unwired: 6 in, 1 out]
